vi "UI Event-Maximize-Value Change.vi"(8 "Error In":errorcluster, 11 "Appearance Actor in":refnum<class "Appearance Actor.lvclass">) -> (0 "Error Out":errorcluster, 3 "Appearance Actor out":refnum<class "Appearance Actor.lvclass">)   [LabVIEW 2021, in "Appearance Actor.lvlib" / "Appearance Actor.lvclass"]
doc: "Handles Maximize Event. By Default, maximizes (or un-maximize if maximized) the FP Window if possible (else return an error). Override this method to change its behavior."
uses:
  Appearance Actor.lvclass
  Appearance Actor.lvclass/Appearance Actor.ctl
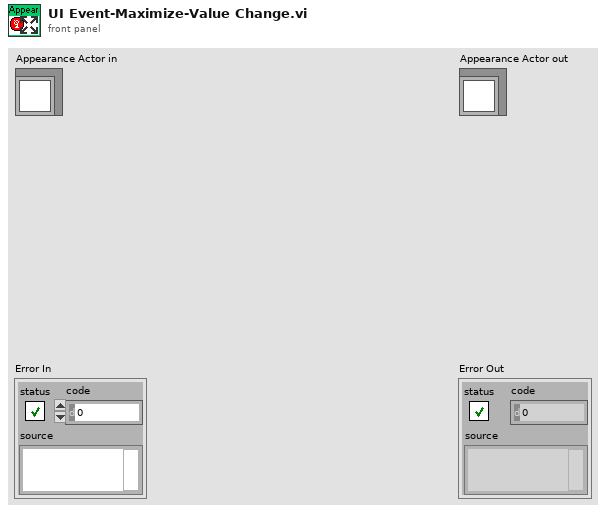
[diagram p1: front panel]
types:
  T1 = enum32{"Invalid", "Standard", "Closed", "Hidden", "Minimized", "Maximized"}
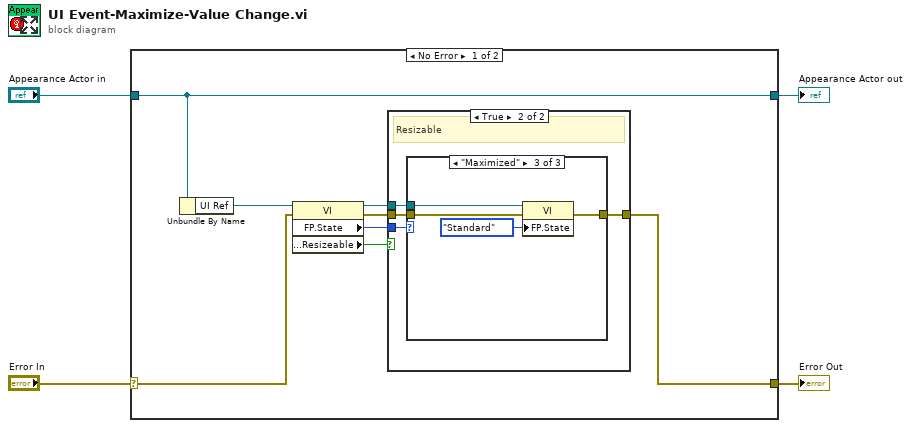
[diagram p0: block diagram]
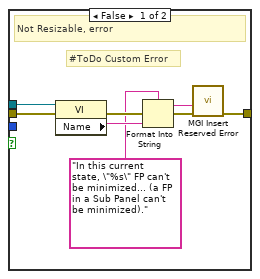
[diagram p2: hidden frame]
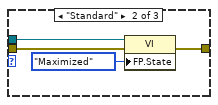
[diagram p4: hidden frame]
diagram:
  n1 = case shown="No Error" "Error In" {
    selector: "Error In" -> [w11 w35]
    tunnel: [w5 w35] -> w3
    tunnel: [w10 w34] -> w1
    tunnel: "Appearance Actor in" -> [w10 w34]
    frame No Error {
      n2 = Unbundle By Name(w10) -> ("UI Ref"=w12:refnum<vi>)
      n3 = property class="VI"(reference=w12, error in=w11) -> (reference out=w9:refnum<vi>, error out=w8:errorcluster, "FP.State"=w7:T1, "Front Panel.Resizeable"=w6:bool)
      n4 = case shown="True" w6 {
        tunnel: w8 -> [w18 w21]
        tunnel: w9 -> [w19 w22]
        tunnel: [w20 w24] -> w5
        tunnel: w7 -> [_ w23]
        frame False {
          # "#ToDo Custom Error"
          # "Not Resizable, error"
          n5 = property class="VI"(reference=w19, error in=w18) -> (error out=w15:errorcluster, "Name"=w14:string)  [unwired: 1 out]
          n6 = Format Into String(format string="In this current state, \"%s\" FP can't be minimized... (a FP in a Sub Panel can't be minimized)." ("Error Description"), error in=w15, w14) -> (resulting string=w17:string, error out=w16:errorcluster)  [unwired: 1 in]
          n7 = call <userlib>:"MGI Insert Reserved Error.vi"("Error In"=w16, "Error Description"=w17) -> ("Error Out"=w20:errorcluster)  [unwired: 9 in]
        }
        frame True {
          # "Resizable"
          n8 = case shown="\"Maximized\"" w23 {
            tunnel: w21 -> [w25 w28 w32]
            tunnel: w22 -> [_ w29 w33]
            tunnel: [w25 w26 w30] -> w24
            frame Default {
              # "#ToDo Error?"
            }
            frame "Standard" {
              n9 = property class="VI"(reference=w29, error in=w28, "FP.State"=T1."Maximized" ("Front Panel Window:State")) -> (error out=w26:errorcluster)  [unwired: 1 out]
            }
            frame "Maximized" {
              n10 = property class="VI"(reference=w33, error in=w32, "FP.State"=T1."Standard" ("Front Panel Window:State")) -> (error out=w30:errorcluster)  [unwired: 1 out]
            }
          }
        }
      }
    }
    frame Error {
    }
  }
  "Error Out" <- w3
  "Appearance Actor out" <- w1
